vi "Rs232_Read-v2.vi"() -> ()   [LabVIEW 2018]
uses:
  <vilib>/Instr/_visa.llb/VISA Configure Serial Port (Instr).vi
panel:
  out "Waveform Chart":dbl(graph)
  out "number":dbl
  in  "stop":bool
  out "error out":errorcluster
  in  "VISA resource name":refnum<visa-resource-name>
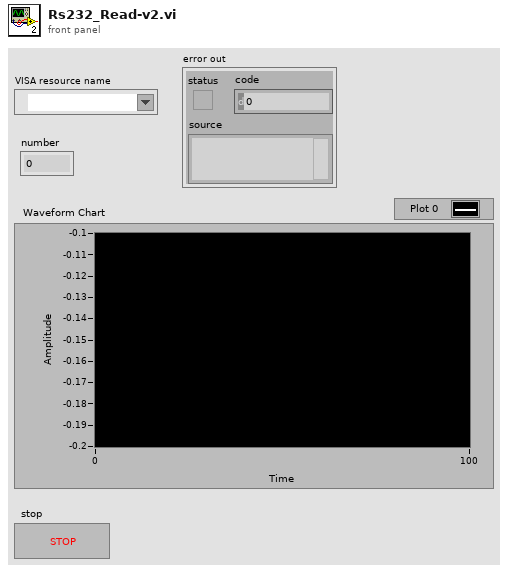
[diagram p1: front panel]
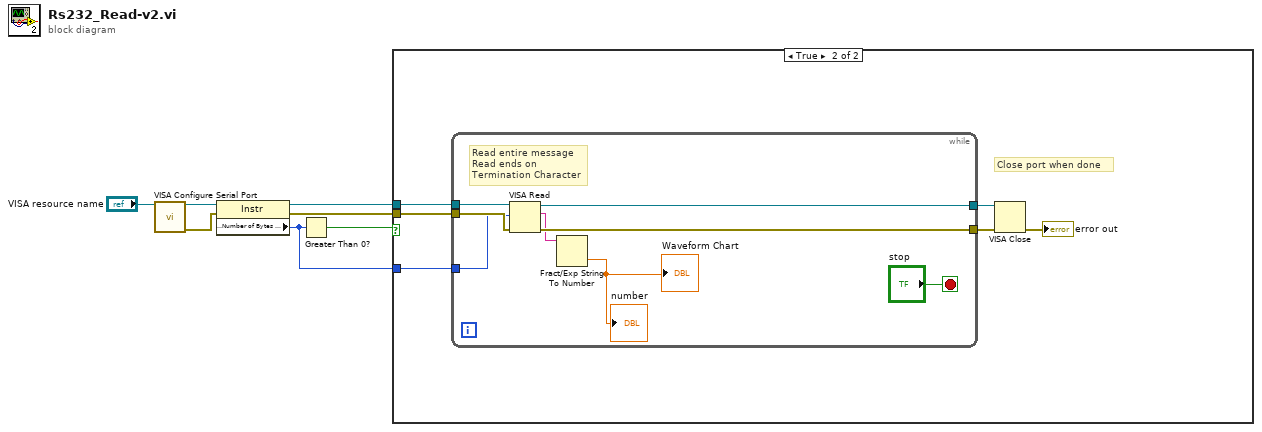
[diagram p0: block diagram]
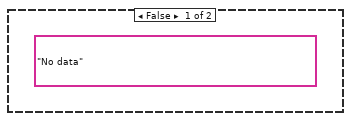
[diagram p2: hidden frame]
diagram:
  n1 = call-poly "VISA Configure Serial Port"("VISA resource name"="VISA resource name") -> ("VISA resource name out"=w6:refnum<visa-resource-name>, "error out"=w5:errorcluster)  [unwired: 13 in]
  n2 = property class="Instr"(reference=w6, error in=w5) -> (reference out=w3:refnum<visa-resource-name>, error out=w2:errorcluster, "Serial Settings:Number of Bytes at Serial Port"=w1:u32)
  n3 = Greater Than 0?(x=w1) -> (x > 0?=w4:bool)
  n4 = case shown="True" w4 {
    tunnel: w3 -> [_ w10]
    tunnel: w2 -> [_ w9]
    tunnel: w1 -> [_ w8]
    frame False {
      (unwired) "No data"
    }
    frame True {
      # "Close port when done"
      n5 = while {
        tunnel: [w20] -> w12
        tunnel: [w19] -> w11
        tunnel: w10 -> [w16]
        tunnel: w9 -> [w15]
        tunnel: w8 -> [w14]
        stop <- "stop" stop-if-true
        # "Read entire message\nRead ends on\nTermination Character"
        n6 = VISA Read(VISA resource name=w16, byte count=w14, error in (no error)=w15) -> (VISA resource name out=w20:refnum<visa-resource-name>, read buffer=w18:string, error out=w19:errorcluster)  [unwired: 1 out]
        n7 = Fract/Exp String To Number(string=w18) -> (number=→"number" →"Waveform Chart":dbl)  [unwired: 3 in, 1 out]
      }
      n8 = VISA Close(VISA resource name=w12, error in (no error)=w11) -> (error out=→"error out":errorcluster)
    }
  }
